vi "POST InspectionSystemsTable.vi"(8 "error in (no error)":errorcluster, 11 "GTron in":path) -> (0 "error out":errorcluster, 3 "DB is Empty?":bool)   [LabVIEW 2015]
uses:
  <vilib>/drjdpowell/SQLite Library/SQL Statement/SQL Statement.lvclass/SQL Statement.ctl
  <vilib>/drjdpowell/SQLite Library/SQL Connection/Open (path).vi
  <vilib>/drjdpowell/SQLite Library/SQL Connection/Open (string).vi
  <vilib>/AdvancedString/Path To Command Line String.vi
  <vilib>/drjdpowell/SQLite Library/SQL Connection/Execute SQL (Single Integer).vi
  <vilib>/drjdpowell/SQLite Library/SQL Statement/Error Message.vi
  <vilib>/drjdpowell/SQLite Library/SQL Statement/Column String.vi
  <vilib>/httpClient/POSTBuffer.vi
  <vilib>/drjdpowell/SQLite Library/SQL Connection/Execute SQL (No results).vi
  <vilib>/drjdpowell/SQLite Library/SQL Connection/Connection.lvclass
  <vilib>/drjdpowell/SQLite Library/SQLite.lvlib
  <vilib>/drjdpowell/SQLite Library/SQL Statement/SQL Statement.lvclass
  DataLogger.lvclass
  <vilib>/httpClient/LabVIEWHTTPClient.lvlib
panel:
  in  "Measurement Keys in":string[](array[string])=["InspectionMcId", "ClientId", "Location", "IotEnable", "SMSAlertEnable", "EmailAlertEnable"]
  in  "Server info Cluster for Measurement in":T1={"JSON Buffer"="authtoken=47244d7c61d7e6141acdddeabbf622d1&scope=creatorapi&zc_ownername=zentron3&XMLString=", "Server information start tag"="<ZohoCreator> <applicationlist> <application name='iiot-gtron'><formlist>  <form name='InspectionSystemsTable'>", "Record start/end"="add", "Key name"="field name", "Value name"="value", "Server information end tag"="\"</form></formlist></application></applicationlist></ZohoCreator>"}
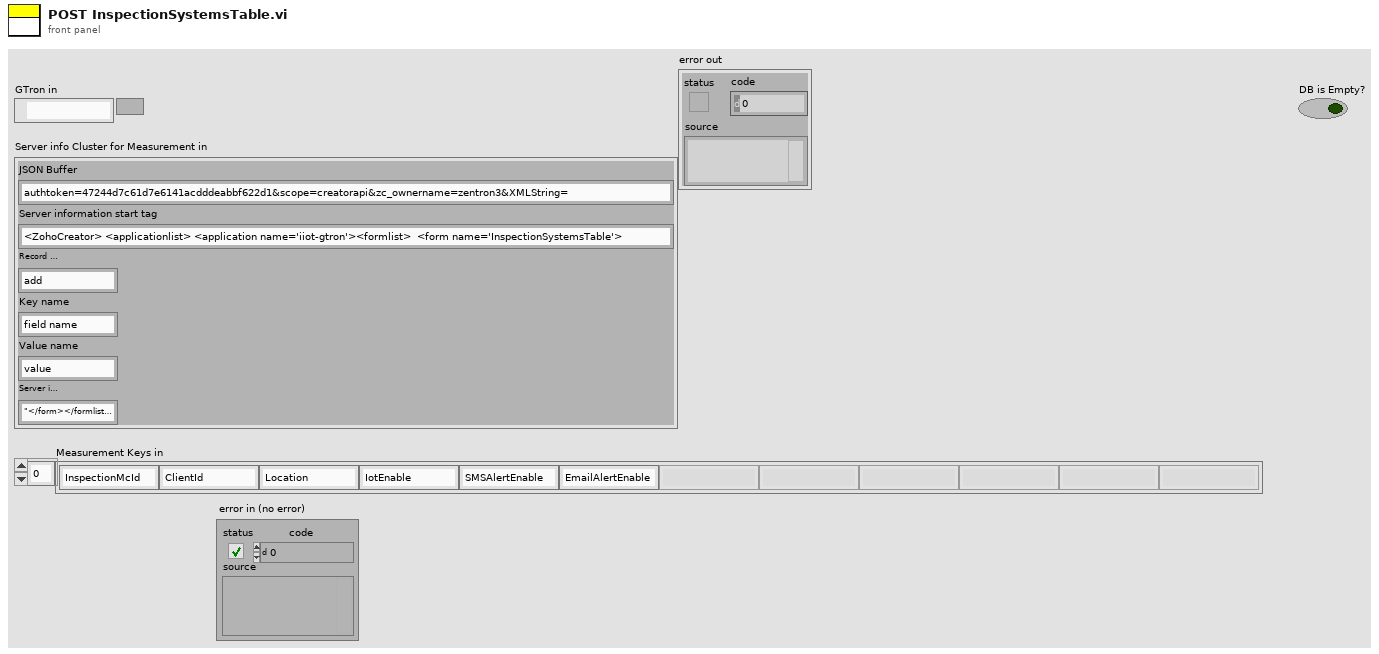
[diagram p1: front panel]
types:
  T1 = cluster{"JSON Buffer":string, "Server information start tag":string, "Record start/end":string, "Key name":string, "Value name":string, "Server information end tag":string}
  T2 = typedef "LabVIEWHTTPClient.lvlib/ClientHandle.ctl" = refnum<k1>
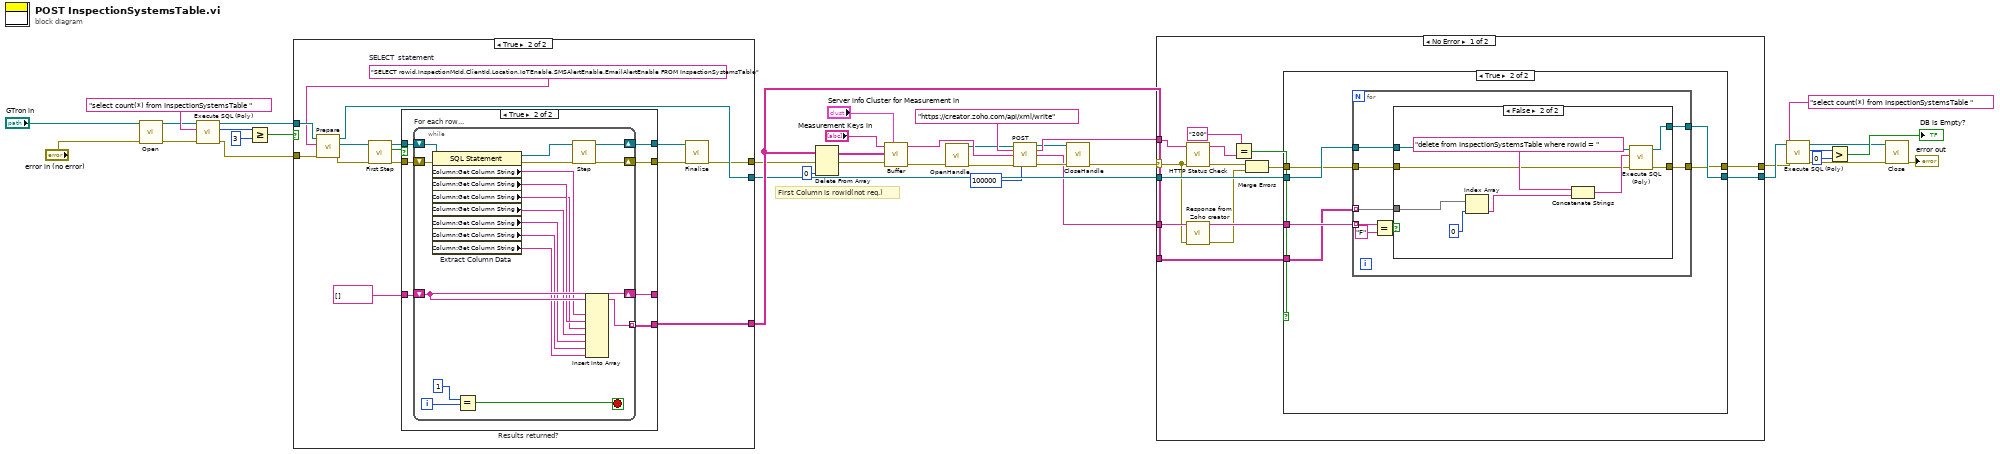
[diagram p0: block diagram]
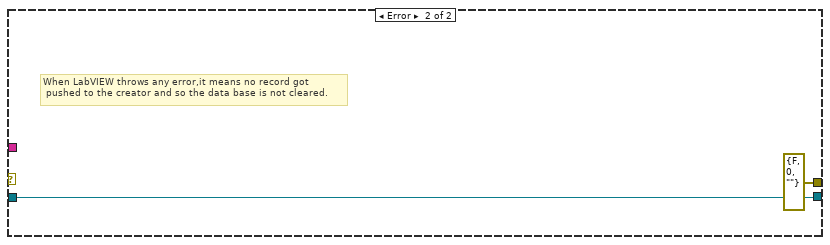
[diagram p4: hidden frame]
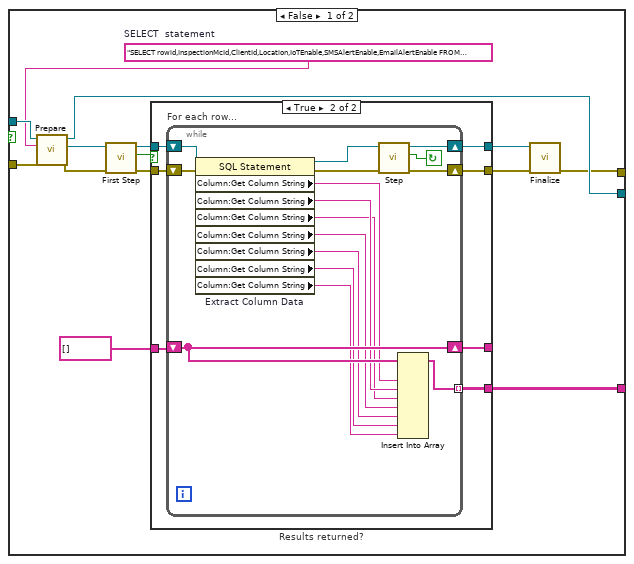
[diagram p5: hidden frame]
diagram:
  # "First Column is rowid(not req.)"
  n1 = call-poly <vilib>:"Open.vi"("error in (no error)"="error in (no error)", "db file"="GTron in") -> ("error out"=w8:errorcluster, "SQLite Connection"=w10:refnum<class "Connection.lvclass">)  [unwired: 8 in]
  n2 = call-poly <vilib>:"Execute SQL (Poly).vi"("error in (no error)"=w8, "SQL"="select count(*) from InspectionSystemsTable ", "SQLite Connection in"=w10) -> ("error out"=w7:errorcluster, "Result"=w12:i64, "SQLite Connection"=w28:refnum<class "Connection.lvclass">)  [unwired: 6 in]
  n3 = Greater Or Equal?(x=w12, y=i64 3) -> (x >= y?=w14:bool)
  n4 = case shown="True" w14 {
    tunnel: [w43 w82] -> w30
    tunnel: w28 -> [w42 w81]
    tunnel: [w41 w80] -> w29
    tunnel: w7 -> [w40 w79]
    tunnel: [w39 w78] -> w6
    frame False {
      w38 = "SELECT rowid,InspectionMcId,ClientId,Location,IoTEnable,SMSAlertEnable,EmailAlertEnable FROM InspectionSystemsTable"  # SELECT  statement
      n5 = call <vilib>:"Prepare.vi"("error in (no error)"=w40, "SQL"=w38, "SQLite Connection in"=w42) -> ("error out"=w50:errorcluster, "SQL Statement"=w46:refnum<class "SQL Statement.lvclass">, "SQLite Connection"=w41:refnum<class "Connection.lvclass">)  [unwired: 4 in, 2 out]
      n6 = call <vilib>:"First Step.vi"("error in (no error)"=w50, "SQL Statement in"=w46) -> ("error out"=w48:errorcluster, "Row returned"=w49:bool, "SQL Statement"=w47:refnum<class "SQL Statement.lvclass">)  [unwired: 7 in]
      n7 = case "Results returned?" shown="True" w49 {
        tunnel: [w53 w60] -> w45
        tunnel: [w52 w59] -> w44
        tunnel: w47 -> [w53 w58]
        tunnel: w48 -> [w52 w57]
        tunnel: string[] [] -> [_ w56]
        tunnel: [_ w55] -> w43
        tunnel: [_ w54] -> _
        frame False {
        }
        frame True {
          n8 = while "For each row..." {
            shift-right: [w75] -> w60
            shift-left: w58 -> [w72]
            shift-right: [w73] -> w59
            shift-left: w57 -> [w71]
            shift-right: [w70] -> w54
            shift-left: w56 -> [w70]
            tunnel: [w63] -> w55 mode=indexing
            stop <- w61 continue-if-true
            n9 = property on="Extract Column Data" class="SQL Statement"(reference=w72, error in=w71) -> (reference out=w76:refnum<class "SQL Statement.lvclass">, error out=w74:errorcluster, "Column:Get Column String"=w62:string, "Column:Get Column String"=w69:string, "Column:Get Column String"=w68:string, "Column:Get Column String"=w67:string, "Column:Get Column String"=w66:string, "Column:Get Column String"=w65:string, "Column:Get Column String"=w64:string)
            n10 = call <vilib>:"Step.vi"("error in (no error)"=w74, "SQL Statement in"=w76) -> ("error out"=w73:errorcluster, "Row returned"=w61:bool, "SQL Statement"=w75:refnum<class "SQL Statement.lvclass">)  [unwired: 7 in]
            n11 = Insert Into Array(array=w70, new element #1=w62, new element #2=w69, new element #3=w68, new element #4=w67, new element #5=w66, new element #6=w65, new element #7=w64) -> (w63:string[])  [unwired: 1 in]
          }
        }
      }
      n12 = call <vilib>:"Finalize.vi"("error in (no error)"=w44, "SQL Statement in"=w45) -> ("error out"=w39:errorcluster)  [unwired: 9 in]
    }
    frame True {
      w77 = "SELECT rowid,InspectionMcId,ClientId,Location,IoTEnable,SMSAlertEnable,EmailAlertEnable FROM InspectionSystemsTable"  # SELECT  statement
      n13 = call <vilib>:"Prepare.vi"("error in (no error)"=w79, "SQL"=w77, "SQLite Connection in"=w81) -> ("error out"=w89:errorcluster, "SQL Statement"=w85:refnum<class "SQL Statement.lvclass">, "SQLite Connection"=w80:refnum<class "Connection.lvclass">)  [unwired: 4 in, 2 out]
      n14 = call <vilib>:"First Step.vi"("error in (no error)"=w89, "SQL Statement in"=w85) -> ("error out"=w87:errorcluster, "Row returned"=w88:bool, "SQL Statement"=w86:refnum<class "SQL Statement.lvclass">)  [unwired: 7 in]
      n15 = case "Results returned?" shown="True" w88 {
        tunnel: [w92 w99] -> w84
        tunnel: [w91 w98] -> w83
        tunnel: w86 -> [w92 w97]
        tunnel: w87 -> [w91 w96]
        tunnel: string[] [] -> [_ w95]
        tunnel: [_ w94] -> w82
        tunnel: [_ w93] -> _
        frame False {
        }
        frame True {
          n16 = while "For each row..." {
            shift-right: [w116] -> w99
            shift-left: w97 -> [w113]
            shift-right: [w114] -> w98
            shift-left: w96 -> [w112]
            shift-right: [w111] -> w93
            shift-left: w95 -> [w111]
            tunnel: [w104] -> w94 mode=indexing
            i -> [w103]
            stop <- w101 stop-if-true
            n17 = property on="Extract Column Data" class="SQL Statement"(reference=w113, error in=w112) -> (reference out=w117:refnum<class "SQL Statement.lvclass">, error out=w115:errorcluster, "Column:Get Column String"=w100:string, "Column:Get Column String"=w110:string, "Column:Get Column String"=w109:string, "Column:Get Column String"=w108:string, "Column:Get Column String"=w107:string, "Column:Get Column String"=w106:string, "Column:Get Column String"=w105:string)
            n18 = Equal?(x=1, y=w103) -> (x = y?=w101:bool)
            n19 = call <vilib>:"Step.vi"("error in (no error)"=w115, "SQL Statement in"=w117) -> ("error out"=w114:errorcluster, "SQL Statement"=w116:refnum<class "SQL Statement.lvclass">)  [unwired: 7 in, 1 out]
            n20 = Insert Into Array(array=w111, new element #1=w100, new element #2=w110, new element #3=w109, new element #4=w108, new element #5=w107, new element #6=w106, new element #7=w105) -> (w104:string[])  [unwired: 1 in]
          }
        }
      }
      n21 = call <vilib>:"Finalize.vi"("error in (no error)"=w83, "SQL Statement in"=w84) -> ("error out"=w78:errorcluster)  [unwired: 9 in]
    }
  }
  n22 = Delete From Array(array=w30, index (col)=0 ("disabled index (col)")) -> (array with subset deleted=w16:string[][])  [unwired: 2 in, 1 out]
  n23 = call "Buffer.vi"("Cluster"="Server info Cluster for Measurement in", "error in"=w6, "Values"=w16, "Keys"="Measurement Keys in") -> ("Error out"=w5:errorcluster, "Buffer"=w21:string)  [unwired: 6 in]
  n24 = call <vilib>:"OpenHandle.vi"("error in (no error)"=w5) -> ("client handle out"=w19:T2, "error out"=w24:errorcluster)  [unwired: 13 in]
  n25 = call-poly <vilib>:"POST.vi"("client handle"=w19, "url"="https://creator.zoho.com/api/xml/write", "buffer"=w21, "error in (no error)"=w24, "timeout (10000)"=100000) -> ("client handle out"=w20:T2, "headers"=w27:string, "body"=w4:string, "error out"=w25:errorcluster)  [unwired: 7 in]
  n26 = call <vilib>:"CloseHandle.vi"("client handle"=w20, "error in (no error)"=w25) -> ("error out"=w26:errorcluster)  [unwired: 13 in]
  n27 = case shown="No Error" w26 {
    selector: w26 -> [w122 _]
    tunnel: w27 -> [w131 _]
    tunnel: w4 -> [w124 _]
    tunnel: w29 -> [w127 w160]
    tunnel: w30 -> [w126 _]
    tunnel: [w125 w160] -> w32
    tunnel: [w118 errorcluster {"status"=FALSE, "code"=0, "source"=""} ("error out")] -> w3
    frame No Error {
      n28 = call "HTTP Status Check.vi"("error in (no error)"=w122, "String"=w131) -> ("error out"=w121:errorcluster, "HTTP Status Code"=w130:string)  [unwired: 7 in]
      n29 = call "Response from Zoho creator.vi"("error in"=w122, "body"=w124) -> ("error out"=w120:errorcluster, "decimated array"=w123:string[])  [unwired: 8 in]
      n30 = Equal?(x="200" ("y"), y=w130) -> (x = y?=w128:bool)
      n31 = Merge Errors(w121, w120) -> (w119:errorcluster)
      n32 = case shown="True" w128 {
        tunnel: w123 -> [_ w138]
        tunnel: w127 -> [w133 w139]
        tunnel: w126 -> [_ w137]
        tunnel: [w133 w136] -> w125
        tunnel: w119 -> [w132 w135]
        tunnel: [w132 w134] -> w118
        frame False {
          # "When HTTP Status is anything except 200,it means no record\ngot pushed to the creator and so the database is not cleared"
        }
        frame True {
          n33 = for {
            tunnel: w139 -> [w147]
            tunnel: w137 -> [w143] mode=indexing
            tunnel: w138 -> [w146] mode=indexing
            tunnel: [w142] -> w136
            tunnel: w135 -> [w141]
            tunnel: [w140] -> w134
            n34 = Equal?(x=w146, y="F") -> (x = y?=w144:bool)
            n35 = case shown="False" w144 {
              tunnel: w147 -> [w149 w158]
              tunnel: w143 -> [_ w157]
              tunnel: [w149 w152] -> w142
              tunnel: w141 -> [w148 w151]
              tunnel: [w148 w150] -> w140
              frame True {
              }
              frame False {
                n36 = Index Array(array=w157, index=0) -> (element=w155:string)
                n37 = Concatenate Strings("delete from InspectionSystemsTable where rowid = " ("SQL"), w155) -> (w153:string)
                n38 = call-poly <vilib>:"Execute SQL (Poly).vi"("error in (no error)"=w151, "SQL"=w153, "SQLite Connection in"=w158) -> ("error out"=w150:errorcluster, "SQLite Connection"=w152:refnum<class "Connection.lvclass">)  [unwired: 7 in]
              }
            }
          }
        }
      }
    }
    frame Error {
      # "When LabVIEW throws any error,it means no record got\n pushed to the creator and so the data base is not cleared."
    }
  }
  n39 = call-poly <vilib>:"Execute SQL (Poly).vi"("error in (no error)"=w3, "SQL"="select count(*) from InspectionSystemsTable ", "SQLite Connection in"=w32) -> ("error out"=w2:errorcluster, "Result"=w33:i64, "SQLite Connection"=w35:refnum<class "Connection.lvclass">)  [unwired: 6 in]
  n40 = Greater?(x=w33, y=i64 0) -> (0:→"DB is Empty?":bool)
  n41 = call-dynamic "Close.vi"("error in (no error)"=w2, "SQLite Connection in"=w35) -> ("error out"=→"error out":errorcluster)  [unwired: 9 in]
